vi "Initialize with Switch Parameters Core.vi"(8 "error in (no error)":errorcluster, 10 "Switch Parameters in":refnum<class "Abstract Switch Init Parameters.lvclass">, 11 "%DEVICE% Consumer in":refnum<class "%DEVICE% Consumer.lvclass">) -> (0 "error out":errorcluster, 3 "%DEVICE% Consumer out":refnum<class "%DEVICE% Consumer.lvclass">)   [LabVIEW 2017, in "%DEVICE% Messaging.lvlib" / "%DEVICE% Consumer.lvclass"]
uses:
  %DEVICE% Consumer.lvclass
  Includes/CDMessaging.lvlibp/Switch/Abstract Switch Init Parameters/Abstract Switch Init Parameters.lvclass
  Session Type.ctl
  %DEVICE% Init Parameters/%DEVICE% Init Parameters.lvclass
  C:/Users/Admin/Documents/niveristand-routing-and-faulting-message-library/Includes/CDMessaging.lvlibp/Switch/Abstract Switch Init Parameters/Abstract Switch Init Parameters.lvclass
  %DEVICE% Consumer.lvclass/%DEVICE% Consumer.ctl
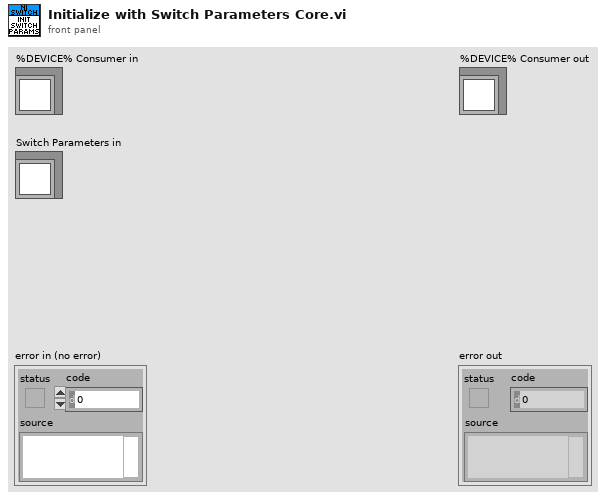
[diagram p1: front panel]
types:
  T1 = typedef "%DEVICE% Messaging.lvlib/%DEVICE% Consumer.lvclass/Session Type.ctl" = picture
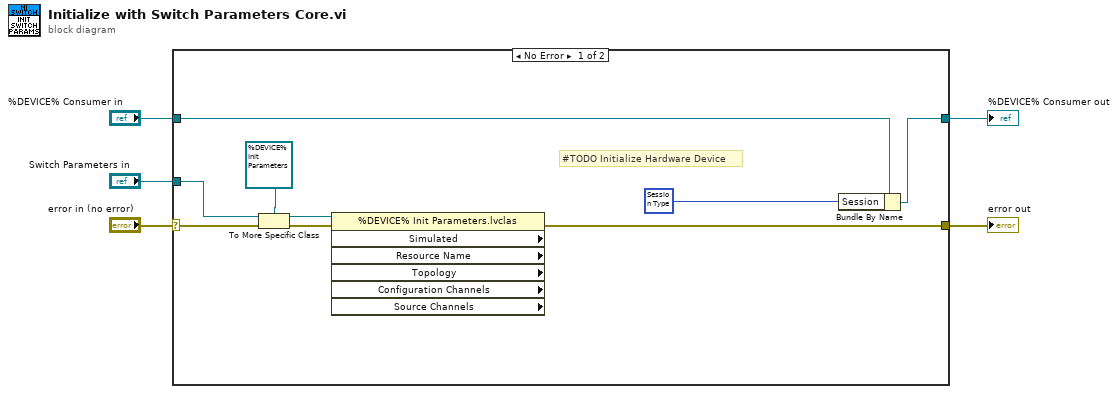
[diagram p0: block diagram]
diagram:
  n1 = case shown="No Error" "error in (no error)" {
    selector: "error in (no error)" -> [w10 w16]
    tunnel: [w8 w16] -> w4
    tunnel: [w13 w15] -> w1
    tunnel: "%DEVICE% Consumer in" -> [w14 w15]
    tunnel: "Switch Parameters in" -> [w12 _]
    frame No Error {
      # "#TODO Initialize Hardware Device"
      n2 = To More Specific Class(target class=refnum<class "%DEVICE% Init Parameters.lvclass"> refnum ("%DEVICE% Messaging.lvlib:%DEVICE% Init Parameters.lvclass"), reference=w12, error in=w10) -> (specific class reference=w11:refnum<class "%DEVICE% Init Parameters.lvclass">, error out=w9:errorcluster)
      n3 = property class="%DEVICE% Init Parameters.lvclas" props=["Simulated", "Resource Name", "Topology", "Configuration Channels", "Source Channels"](reference=w11, error in=w9) -> (error out=w8:errorcluster)  [unwired: 6 out]
      n4 = Bundle By Name(cluster=w14, "Session"=T1 data[5B]) -> (w13:refnum<class "%DEVICE% Consumer.lvclass">)
    }
    frame Error {
    }
  }
  "error out" <- w4
  "%DEVICE% Consumer out" <- w1
